vi "Open Sensors and Actuators.vi"   [LabVIEW 2014]
uses:
  <vilib>/Rock Robotics/SystemInterfaces/DIO/FPGA_DIOPWMChannel.ctl
  <vilib>/Rock Robotics/SystemInterfaces/AI/FPGA_AIChannel.ctl
  <vilib>/Rock Robotics/WPI/Joystick/WPI_JoystickDeviceEnum.ctl
  <vilib>/Rock Robotics/SystemInterfaces/DIO/FPGA_DIOChannel.ctl
  <vilib>/Rock Robotics/WPI/Solenoid/WPI_SolenoidChannel.ctl
  <vilib>/Rock Robotics/SystemInterfaces/Typedef/FPGA_TypedefDigitalModule.ctl
  <vilib>/Rock Robotics/SystemInterfaces/i2clib/i2c_bus.ctl
  <vilib>/Rock Robotics/WPI/MotorControl/WPI_MotorControlOpen Talon.vi
  <vilib>/Rock Robotics/WPI/Counter/WPI_CounterDigitalInputToDigitalSource.vi
  <vilib>/Rock Robotics/WPI/Counter/WPI_CounterOpen UpDown Mode.vi
  <vilib>/Rock Robotics/WPI/Solenoid/WPI_SolenoidOpenSingle.vi
  Global RefNums.vi
  Global Variables.vi
  _Dependencies/NavX/navX-MXP IMU.lvlib
types:
  T1 = typedef "i2c_bus.ctl" = enum16{"I2C On-Board", "I2C MXP", "Invalid"}
  T2 = typedef "FPGA_TypedefDigitalModule.ctl" = enum16{"Controller 1"}
  T3 = typedef "WPI_SolenoidChannel.ctl" = enum8{"Solenoid 0", "Solenoid 1", "Solenoid 2", "Solenoid 3", "Solenoid 4", "Solenoid 5", "Solenoid 6", "Solenoid 7", "Invalid"}
  T4 = typedef "FPGA_DIOPWMChannel.ctl" = enum8{"PWM 0", "PWM 1", "PWM 2", "PWM 3", "PWM 4", "PWM 5", "PWM 6", "PWM 7", "PWM 8", "PWM 9", "PWM MXP 0", "PWM MXP 1", "PWM MXP 2", "PWM MXP 3", "PWM MXP 4", "PWM MXP 5", "PWM MXP 6", "PWM MXP 7", "PWM MXP 8", "PWM MXP 9", "Invalid"}
  T5 = typedef "FPGA_DIOChannel.ctl" = enum8{"DIO 0", "DIO 1", "DIO 2", "DIO 3", "DIO 4", "DIO 5", "DIO 6", "DIO 7", "DIO 8", "DIO 9", "DIO MXP 0", "DIO MXP 1", "DIO MXP 2", "DIO MXP 3", "DIO MXP 4", "DIO MXP 5", "DIO MXP 6", "DIO MXP 7", "DIO MXP 8", "DIO MXP 9", "DIO MXP 10", "DIO MXP 11", "DIO MXP 12", "DIO MXP 13", "DIO MXP 14", "DIO MXP 15", "Invalid"}
  T6 = typedef "WPI_JoystickDeviceEnum.ctl" = enum16{"USB 0", "USB 1", "USB 2", "USB 3", "USB 4", "USB 5"}
  T7 = typedef "FPGA_AIChannel.ctl" = enum8{"AI 0", "AI 1", "AI 2", "AI 3", "AI MXP 0", "AI MXP 1", "AI MXP 2", "AI MXP 3", "Invalid"}
  T8 = typedef "WPI_MotorControlDeviceRef.ctl" = cluster{"DeviceStatus":errorcluster, "Type":T9, "PWM":cluster{"Controller":T2, "PWM Channel":T4, "DeadBand":T10}, "CAN":cluster{"Device Number":u8, "Control Mode":T11, "Semaphore":T12, "Max Vout":dbl, "TalonSRX Control Mode":T13}, "Invert":bool, "TransformRef":T14, "InvTransformRef":T14}
  T9 = typedef "WPI_MotorControlType.ctl" = enum16{"PWM", "CAN", "CANTalonSRX"}
  T10 = typedef "WPI_PWMDeadband.ctl" = cluster{"Name":string, "maxPositivePwm":i32, "minPositivePwm":i32, "centerPwm":i32, "maxNegativePwm":i32, "minNegativePwm":i32, "angularRange":u16}
  T11 = typedef "WPI_CANJaguar_ControlMode.ctl" = enum8{"Percent VBus", "Current", "Speed", "Position", "Voltage"}
  T12 = typedef "Semaphore RefNum" = refnum<k1>
  T13 = typedef "WPI_CANTalonSRX_APIControlMode.ctl" = enum8{"Percent VBus", "Speed", "Position", "Slave", "Unchanged / Invalid"}
  T14 = typedef "WPI_PWMTransform_ConPane.ctl" = refnum<vi>
  T15 = typedef "WPI_DigitalInputDevRef.ctl" = cluster{"DevStatus":errorcluster, "DIO Channel":T5, "Controller":T2}
  T16 = typedef "FPGA_CounterEncoderSourceConvertionLVSourceType.ctl" = cluster{"DevStatus":errorcluster, "AnalogTriggerMode?":bool, "DigitalMode":cluster{"Controller":T2, "DIO Channel":T17}, "AnalogTriggerMode":cluster{"AnalogTriggerIndex":T18, "OutputType":T19}}
  T17 = typedef "FPGA_DIODigitalSourceChannel.ctl" = enum8{"DIO 0", "DIO 1", "DIO 2", "DIO 3", "DIO 4", "DIO 5", "DIO 6", "DIO 7", "DIO 8", "DIO 9", "DIO MXP 0", "DIO MXP 1", "DIO MXP 2", "DIO MXP 3", "DIO MXP 4", "DIO MXP 5", "DIO MXP 6", "DIO MXP 7", "DIO MXP 8", "DIO MXP 9", "DIO MXP 10", "DIO MXP 11", "DIO MXP 12", "DIO MXP 13", "DIO MXP 14", "DIO MXP 15", "Disabled"}
  T18 = typedef "FPGA_AnalogTriggerIndex.ctl" = enum8{"Trig 0", "Trig 1", "Trig 2", "Trig 3", "Trig 4", "Trig 5", "Trig 6", "Trig 7", "Invalid"}
  T19 = typedef "FPGA_AnalogTriggerOutType.ctl" = enum16{"InWindow", "TriggerState", "Rising", "Falling"}
  T20 = typedef "WPI_EncoderDevRef.ctl" = cluster{"DevStatus":errorcluster, "EncoderIndex":T21, "CounterIndex":T22, "DistancePerCount":dbl, "Decoding Type":T23}
  T21 = typedef "FPGA_EncoderIdx.ctl" = enum8{"Enc 0", "Enc 1", "Enc 2", "Enc 3", "Enc 4", "Enc 5", "Enc 6", "Enc 7", "Invalid"}
  T22 = typedef "FPGA_CounterCtrSystemIndex.ctl" = enum8{"Ctr 0", "Ctr 1", "Ctr 2", "Ctr 3", "Ctr 4", "Ctr 5", "Ctr 6", "Ctr 7", "Invalid"}
  T23 = typedef "WPI_EncoderType.ctl" = enum16{"1x", "2x", "4x"}
  T24 = typedef "WPI_JoystickDevRef.ctl" = cluster{"Device":T6}
  T25 = typedef "WPI_AnalogChannelDevRef.ctl" = cluster{"DevStatus":errorcluster, "Controller":T26, "Analog Channel":T7}
  T26 = typedef "FPGA_TypedefAnalogModule.ctl" = enum16{"Controller 1"}
  T27 = typedef "WPI_SolenoidDevRef.ctl" = cluster{"DevStatus":errorcluster, "Pneumatics Control Module":u8, "Forward Solenoid Channel":T3, "Reverse Solenoid Channel":T3}
  T28 = typedef "navX-MXP IMU.lvlib/navX Device TypeDef.ctl" = cluster{"navX Interface Protocol":T29, "navX Interface Protocol TypeDefs":cluster{"SPIDevRef":T30, "I2CDevRef":T32}, "navX System Information":cluster{"Board Information":T33, "Status":T34, "Offsets":T38}, "navX Common Information":cluster{"Update Rate (4Hz-60Hz)":T39, "refnum name":string, "error":errorcluster}}
  T29 = typedef "navX-MXP IMU.lvlib/navX Interface Protocol.ctl" = enum16{"SPI", "I2C"}
  T30 = typedef "WPI_SPIDevRef.ctl" = cluster{"DevStatus":errorcluster, "Handle":i32, "Controller":T2, "SPI Bus":T31}
  T31 = typedef "spi_bus.ctl" = enum16{"SPI On-Board, CS0", "SPI On-Board, CS1", "SPI On-Board, CS2", "SPI On-Board, CS3", "SPI MXP", "Invalid"}
  T32 = typedef "WPI_I2CDevRef.ctl" = cluster{"DevStatus":errorcluster, "Controller":T2, "Device Address":u8, "Handle":i32, "I2C Bus":T1}
  T33 = typedef "navX-MXP IMU.lvlib/navX Board Information.ctl" = cluster{"WhoAmI (50 | 0x32)":u8, "Board Revision":u8, "Firmware Major Version":u8, "Firmware Minor Version":u8}
  T34 = typedef "navX-MXP IMU.lvlib/navX Status Data.ctl" = cluster{"Update Rate Hz":u8, "Accelerometer Full-Scale Range":u8, "Gyro Full-Scale Range":u16, "NAVX_OP_STATUS":T35, "NAVX_CAL_STATUS":T36, "NAVX_SELFTEST_STATUS":u8, "NAVX_SENSOR_STATUS":T37}
  T35 = typedef "navX-MXP IMU.lvlib/navX NAVX_OP_STATUS.ctl" = u8
  T36 = typedef "navX-MXP IMU.lvlib/navX NAVX_CAL_STATUS.ctl" = u8
  T37 = typedef "navX-MXP IMU.lvlib/navX NAVX_SENSOR_STATUS.ctl" = cluster{"MOVING":bool, "YAW_STABLE":bool, "MAG_DISTURBANCE":bool, "ALTITUDE_VALID":bool, "SEALEVEL_PRESS_SET":bool, "FUSED_HEADING_VALID":bool}
  T38 = typedef "navX-MXP IMU.lvlib/navX Offsets Data.ctl" = cluster{"Yaw":dbl, "Quat W":dbl, "Quat X":dbl, "Quat Y":dbl, "Quat Z":dbl}
  T39 = typedef "navX-MXP IMU.lvlib/navX Update Rate.ctl" = u8
  T40 = typedef "WPI_CounterDevRef.ctl" = cluster{"DevStatus":errorcluster, "CntIndex":T22}
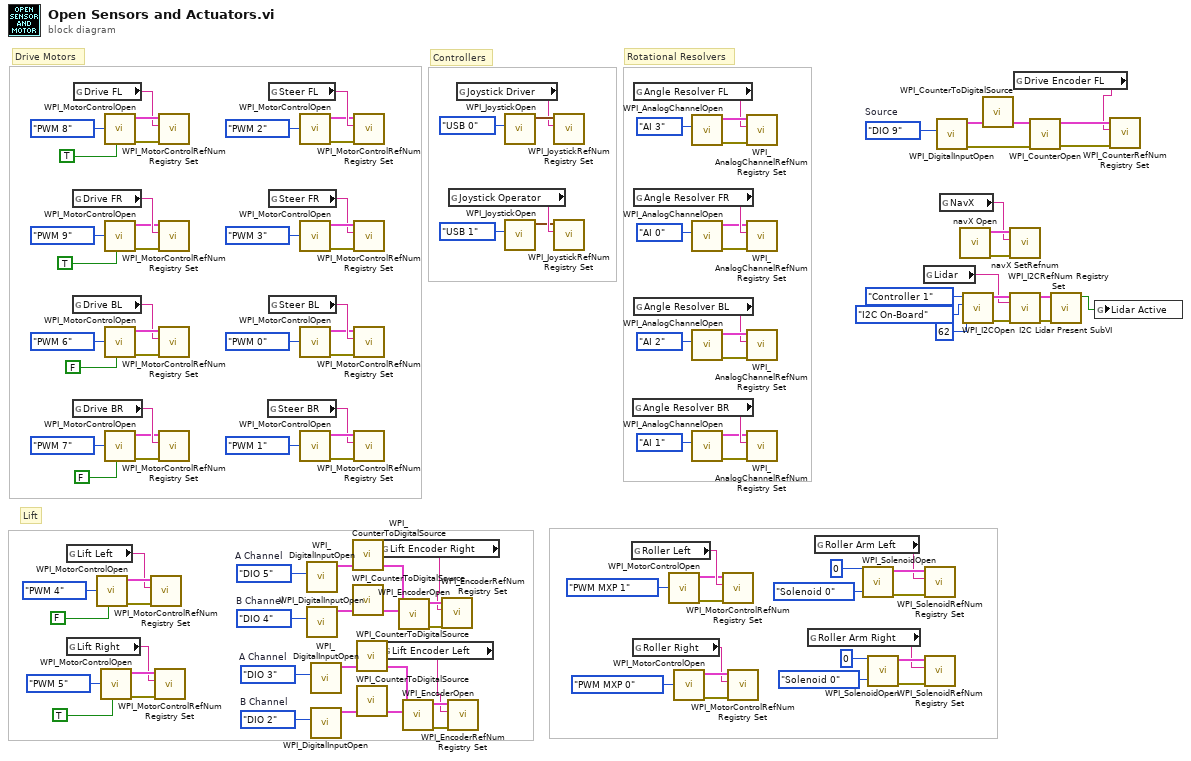
[diagram p0: block diagram]
diagram:
  w41 = FPGA_DIOChannel."DIO 2"  # B Channel
  w40 = FPGA_DIOChannel."DIO 3"  # A Channel
  w47 = FPGA_DIOChannel."DIO 4"  # B Channel
  w46 = FPGA_DIOChannel."DIO 5"  # A Channel
  w68 = FPGA_DIOChannel."DIO 9"  # Source
  # "Lift"
  # "Drive Motors"
  # "Controllers"
  # "Rotational Resolvers"
  n1 = global read "Global RefNums.vi" "Lift Left"() -> (w57:string)
  n2 = global read "Global RefNums.vi" "Lift Right"() -> (w53:string)
  n3 = global read "Global RefNums.vi" "Drive FR"() -> (w115:string)
  n4 = global read "Global RefNums.vi" "Drive BL"() -> (w110:string)
  n5 = global read "Global RefNums.vi" "Drive BR"() -> (w107:string)
  n6 = global read "Global RefNums.vi" "Drive FL"() -> (w118:string)
  n7 = call-poly <vilib>:"WPI_MotorControlOpen.vi"("Invert"=FALSE, "PWM Channel"=FPGA_DIOPWMChannel."PWM 4") -> ("error out"=w58:errorcluster, "MotorControlDeviceRef"=w59:T8)  [unwired: 8 in]
  n8 = call-poly <vilib>:"WPI_MotorControlOpen.vi"("Invert"=TRUE, "PWM Channel"=FPGA_DIOPWMChannel."PWM 5") -> ("error out"=w54:errorcluster, "MotorControlDeviceRef"=w55:T8)  [unwired: 8 in]
  n9 = call-poly <vilib>:"WPI_MotorControlOpen.vi"("Invert"=TRUE, "PWM Channel"=FPGA_DIOPWMChannel."PWM 8") -> ("error out"=w119:errorcluster, "MotorControlDeviceRef"=w120:T8)  [unwired: 8 in]
  n10 = call-poly <vilib>:"WPI_MotorControlOpen.vi"("Invert"=TRUE, "PWM Channel"=FPGA_DIOPWMChannel."PWM 9") -> ("error out"=w114:errorcluster, "MotorControlDeviceRef"=w113:T8)  [unwired: 8 in]
  n11 = call-poly <vilib>:"WPI_MotorControlOpen.vi"("Invert"=FALSE, "PWM Channel"=FPGA_DIOPWMChannel."PWM 6") -> ("error out"=w111:errorcluster, "MotorControlDeviceRef"=w112:T8)  [unwired: 8 in]
  n12 = call-poly <vilib>:"WPI_MotorControlOpen.vi"("Invert"=FALSE, "PWM Channel"=FPGA_DIOPWMChannel."PWM 7") -> ("error out"=w106:errorcluster, "MotorControlDeviceRef"=w105:T8)  [unwired: 8 in]
  n13 = call <vilib>:"WPI_MotorControlRefNum Registry Set.vi"("error in (no error)"=w58, "refnum name"=w57, "MotorControlDevRef"=w59) -> ()  [unwired: 7 in, 2 out]
  n14 = call <vilib>:"WPI_MotorControlRefNum Registry Set.vi"("error in (no error)"=w54, "refnum name"=w53, "MotorControlDevRef"=w55) -> ()  [unwired: 7 in, 2 out]
  n15 = call <vilib>:"WPI_MotorControlRefNum Registry Set.vi"("error in (no error)"=w119, "refnum name"=w118, "MotorControlDevRef"=w120) -> ()  [unwired: 7 in, 2 out]
  n16 = call <vilib>:"WPI_MotorControlRefNum Registry Set.vi"("error in (no error)"=w114, "refnum name"=w115, "MotorControlDevRef"=w113) -> ()  [unwired: 7 in, 2 out]
  n17 = call <vilib>:"WPI_MotorControlRefNum Registry Set.vi"("error in (no error)"=w111, "refnum name"=w110, "MotorControlDevRef"=w112) -> ()  [unwired: 7 in, 2 out]
  n18 = call <vilib>:"WPI_MotorControlRefNum Registry Set.vi"("error in (no error)"=w106, "refnum name"=w107, "MotorControlDevRef"=w105) -> ()  [unwired: 7 in, 2 out]
  n19 = global read "Global RefNums.vi" "Steer BR"() -> (w102:string)
  n20 = global read "Global RefNums.vi" "Steer FL"() -> (w91:string)
  n21 = global read "Global RefNums.vi" "Steer FR"() -> (w94:string)
  n22 = global read "Global RefNums.vi" "Steer BL"() -> (w99:string)
  n23 = call-poly <vilib>:"WPI_MotorControlOpen.vi"("PWM Channel"=FPGA_DIOPWMChannel."PWM 2") -> ("error out"=w90:errorcluster, "MotorControlDeviceRef"=w89:T8)  [unwired: 9 in]
  n24 = call-poly <vilib>:"WPI_MotorControlOpen.vi"("PWM Channel"=FPGA_DIOPWMChannel."PWM 3") -> ("error out"=w95:errorcluster, "MotorControlDeviceRef"=w96:T8)  [unwired: 9 in]
  n25 = call-poly <vilib>:"WPI_MotorControlOpen.vi"("PWM Channel"=FPGA_DIOPWMChannel."PWM 0") -> ("error out"=w98:errorcluster, "MotorControlDeviceRef"=w97:T8)  [unwired: 9 in]
  n26 = call-poly <vilib>:"WPI_MotorControlOpen.vi"("PWM Channel"=FPGA_DIOPWMChannel."PWM 1") -> ("error out"=w103:errorcluster, "MotorControlDeviceRef"=w104:T8)  [unwired: 9 in]
  n27 = call <vilib>:"WPI_DigitalInputOpen.vi"("DIO Channel"=w46) -> ("DigitalInputDevRef"=w43:T15)  [unwired: 2 in, 8 out]
  n28 = call <vilib>:"WPI_DigitalInputOpen.vi"("DIO Channel"=w47) -> ("DigitalInputDevRef"=w44:T15)  [unwired: 2 in, 8 out]
  n29 = call <vilib>:"WPI_DigitalInputOpen.vi"("DIO Channel"=w40) -> ("DigitalInputDevRef"=w37:T15)  [unwired: 2 in, 8 out]
  n30 = call <vilib>:"WPI_DigitalInputOpen.vi"("DIO Channel"=w41) -> ("DigitalInputDevRef"=w38:T15)  [unwired: 2 in, 8 out]
  n31 = call-poly <vilib>:"WPI_CounterToDigitalSource.vi"("DigitalInputDevRef"=w43) -> ("Digital Source"=w42:T16)  [unwired: 6 out]
  n32 = call-poly <vilib>:"WPI_CounterToDigitalSource.vi"("DigitalInputDevRef"=w44) -> ("Digital Source"=w45:T16)  [unwired: 6 out]
  n33 = call <vilib>:"WPI_MotorControlRefNum Registry Set.vi"("error in (no error)"=w90, "refnum name"=w91, "MotorControlDevRef"=w89) -> ()  [unwired: 7 in, 2 out]
  n34 = call <vilib>:"WPI_MotorControlRefNum Registry Set.vi"("error in (no error)"=w95, "refnum name"=w94, "MotorControlDevRef"=w96) -> ()  [unwired: 7 in, 2 out]
  n35 = call <vilib>:"WPI_MotorControlRefNum Registry Set.vi"("error in (no error)"=w98, "refnum name"=w99, "MotorControlDevRef"=w97) -> ()  [unwired: 7 in, 2 out]
  n36 = call <vilib>:"WPI_MotorControlRefNum Registry Set.vi"("error in (no error)"=w103, "refnum name"=w102, "MotorControlDevRef"=w104) -> ()  [unwired: 7 in, 2 out]
  n37 = call-poly <vilib>:"WPI_CounterToDigitalSource.vi"("DigitalInputDevRef"=w37) -> ("Digital Source"=w36:T16)  [unwired: 6 out]
  n38 = call-poly <vilib>:"WPI_CounterToDigitalSource.vi"("DigitalInputDevRef"=w38) -> ("Digital Source"=w39:T16)  [unwired: 6 out]
  n39 = global read "Global RefNums.vi" "Lift Encoder Right"() -> (w30:string)
  n40 = global read "Global RefNums.vi" "Lift Encoder Left"() -> (w31:string)
  n41 = call <vilib>:"WPI_EncoderOpen.vi"("BSource"=w45, "ASource"=w42) -> ("error out"=w35:errorcluster, "EncoderDevRef"=w34:T20)  [unwired: 6 in, 2 out]
  n42 = call <vilib>:"WPI_EncoderOpen.vi"("BSource"=w39, "ASource"=w36) -> ("error out"=w33:errorcluster, "EncoderDevRef"=w32:T20)  [unwired: 6 in, 2 out]
  n43 = call <vilib>:"WPI_EncoderRefNum Registry Set.vi"("error in (no error)"=w35, "refnum name"=w30, "EncoderDevRef"=w34) -> ()  [unwired: 7 in, 2 out]
  n44 = call <vilib>:"WPI_EncoderRefNum Registry Set.vi"("error in (no error)"=w33, "refnum name"=w31, "EncoderDevRef"=w32) -> ()  [unwired: 7 in, 2 out]
  n45 = global read "Global RefNums.vi" "Joystick Operator"() -> (w87:string)
  n46 = global read "Global RefNums.vi" "Joystick Driver"() -> (w88:string)
  n47 = call <vilib>:"WPI_JoystickOpen.vi"("JoystickDevice"=WPI_JoystickDeviceEnum."USB 0") -> ("JoystickDevRef"=w121:T24)  [unwired: 10 in]
  n48 = call <vilib>:"WPI_JoystickOpen.vi"("JoystickDevice"=WPI_JoystickDeviceEnum."USB 1") -> ("JoystickDevRef"=w86:T24)  [unwired: 10 in]
  n49 = call <vilib>:"WPI_JoystickRefNum Registry Set.vi"("refnum name"=w88, "JoystickDevRef"=w121) -> ()  [unwired: 8 in, 2 out]
  n50 = call <vilib>:"WPI_JoystickRefNum Registry Set.vi"("refnum name"=w87, "JoystickDevRef"=w86) -> ()  [unwired: 8 in, 2 out]
  n51 = global read "Global RefNums.vi" "Roller Left"() -> (w26:string)
  n52 = global read "Global RefNums.vi" "Angle Resolver BR"() -> (w74:string)
  n53 = global read "Global RefNums.vi" "Roller Right"() -> (w21:string)
  n54 = global read "Global RefNums.vi" "Angle Resolver FL"() -> (w85:string)
  n55 = global read "Global RefNums.vi" "Angle Resolver FR"() -> (w82:string)
  n56 = global read "Global RefNums.vi" "Angle Resolver BL"() -> (w77:string)
  n57 = call-poly <vilib>:"WPI_MotorControlOpen.vi"("PWM Channel"=FPGA_DIOPWMChannel."PWM MXP 1") -> ("error out"=w25:errorcluster, "MotorControlDeviceRef"=w24:T8)  [unwired: 9 in]
  n58 = call-poly <vilib>:"WPI_MotorControlOpen.vi"("PWM Channel"=FPGA_DIOPWMChannel."PWM MXP 0") -> ("error out"=w22:errorcluster, "MotorControlDeviceRef"=w23:T8)  [unwired: 9 in]
  n59 = call <vilib>:"WPI_AnalogChannelOpen.vi"("Analog Channel"=FPGA_AIChannel."AI 3") -> ("error out"=w123:errorcluster, "AIDeviceRef"=w122:T25)  [unwired: 9 in]
  n60 = call <vilib>:"WPI_AnalogChannelOpen.vi"("Analog Channel"=FPGA_AIChannel."AI 0") -> ("error out"=w80:errorcluster, "AIDeviceRef"=w81:T25)  [unwired: 9 in]
  n61 = call <vilib>:"WPI_AnalogChannelOpen.vi"("Analog Channel"=FPGA_AIChannel."AI 2") -> ("error out"=w79:errorcluster, "AIDeviceRef"=w78:T25)  [unwired: 9 in]
  n62 = call <vilib>:"WPI_AnalogChannelOpen.vi"("Analog Channel"=FPGA_AIChannel."AI 1") -> ("error out"=w72:errorcluster, "AIDeviceRef"=w73:T25)  [unwired: 9 in]
  n63 = call <vilib>:"WPI_MotorControlRefNum Registry Set.vi"("error in (no error)"=w25, "refnum name"=w26, "MotorControlDevRef"=w24) -> ()  [unwired: 7 in, 2 out]
  n64 = call <vilib>:"WPI_MotorControlRefNum Registry Set.vi"("error in (no error)"=w22, "refnum name"=w21, "MotorControlDevRef"=w23) -> ()  [unwired: 7 in, 2 out]
  n65 = call <vilib>:"WPI_AnalogChannelRefNum Registry Set.vi"("error in (no error)"=w123, "refnum name"=w85, "AIDeviceRef"=w122) -> ()  [unwired: 7 in, 2 out]
  n66 = call <vilib>:"WPI_AnalogChannelRefNum Registry Set.vi"("error in (no error)"=w80, "refnum name"=w82, "AIDeviceRef"=w81) -> ()  [unwired: 7 in, 2 out]
  n67 = call <vilib>:"WPI_AnalogChannelRefNum Registry Set.vi"("error in (no error)"=w79, "refnum name"=w77, "AIDeviceRef"=w78) -> ()  [unwired: 7 in, 2 out]
  n68 = call <vilib>:"WPI_AnalogChannelRefNum Registry Set.vi"("error in (no error)"=w72, "refnum name"=w74, "AIDeviceRef"=w73) -> ()  [unwired: 7 in, 2 out]
  n69 = global read "Global RefNums.vi" "Roller Arm Right"() -> (w10:string)
  n70 = global read "Global RefNums.vi" "Roller Arm Left"() -> (w11:string)
  n71 = call-poly <vilib>:"WPI_SolenoidOpen.vi"("Solenoid Channel"=WPI_SolenoidChannel."Solenoid 0", "Pneumatics Control Module (0)"=u8 0) -> ("error out"=w16:errorcluster, "SolenoidDevRef"=w17:T27)  [unwired: 8 in]
  n72 = call-poly <vilib>:"WPI_SolenoidOpen.vi"("Solenoid Channel"=WPI_SolenoidChannel."Solenoid 0", "Pneumatics Control Module (0)"=u8 0) -> ("error out"=w19:errorcluster, "SolenoidDevRef"=w18:T27)  [unwired: 8 in]
  n73 = global read "Global RefNums.vi" "Lidar"() -> (w7:string)
  n74 = call <vilib>:"WPI_SolenoidRefNum Registry Set.vi"("error in (no error)"=w16, "refnum name"=w11, "SolenoidDevRef"=w17) -> ()  [unwired: 7 in, 2 out]
  n75 = call <vilib>:"WPI_SolenoidRefNum Registry Set.vi"("error in (no error)"=w19, "refnum name"=w10, "SolenoidDevRef"=w18) -> ()  [unwired: 7 in, 2 out]
  n76 = call <vilib>:"WPI_DigitalInputOpen.vi"("DIO Channel"=w68) -> ("error out"=w64:errorcluster, "DigitalInputDevRef"=w67:T15)  [unwired: 2 in, 7 out]
  n77 = global read "Global RefNums.vi" "NavX"() -> (w60:string)
  n78 = call "navX Open.vi"() -> ("error out"=w62:errorcluster, "navX Device TypeDef"=w61:T28)  [unwired: 9 in, 1 out]
  n79 = call <vilib>:"WPI_I2COpen.vi"("Device Address"=u8 62, "I2C Bus"=i2c_bus."I2C On-Board", "Controller"=FPGA_TypedefDigitalModule."Controller 1") -> ("error out"=w9:errorcluster, "I2CDevRef"=w8:T32)  [unwired: 7 in]
  n80 = call-poly <vilib>:"WPI_CounterToDigitalSource.vi"("DigitalInputDevRef"=w67) -> ("Digital Source"=w69:T16)  [unwired: 6 out]
  n81 = call "navX SetRefnum.vi"("error in (no error)"=w62, "refnum name"=w60, "navX Device TypeDef"=w61) -> ()  [unwired: 7 in, 2 out]
  n82 = call <vilib>:"WPI_I2CRefNum Registry Set.vi"("error in (no error)"=w9, "refnum name"=w7, "I2CDevRef"=w8) -> ("error out"=w2:errorcluster, "I2CDevRef"=w3:T32)  [unwired: 7 in]
  n83 = global read "Global RefNums.vi" "Drive Encoder FL"() -> (w63:string)
  n84 = call-poly <vilib>:"WPI_CounterOpen.vi"("error in (no error)"=w64, "Up Source"=w69) -> ("error out"=w65:errorcluster, "CounterDevRef"=w66:T40)  [unwired: 5 in, 3 out]
  n85 = call "I2C Lidar Present SubVI.vi"("error in (no error)"=w2, "I2CDevRef"=w3) -> ("Sensor Present"=w1:bool)  [unwired: 9 in]
  n86 = global write "Global Variables.vi" "Lidar Active"(w1) -> ()
  n87 = call <vilib>:"WPI_CounterRefNum Registry Set.vi"("error in (no error)"=w65, "refnum name"=w63, "CounterDevRef"=w66) -> ()  [unwired: 7 in, 2 out]
